vi "Configure Setpoint.vi"   [LabVIEW 2024, in "Bronkhorst FLOW-BUS.lvlib"]
doc: "Configures the setpoint value in the instrument. The setpoint is used to tell the PID controller in the instrument what the wanted amount of mass flow or pressure is."
uses:
  Bronkhorst FLOW-BUS.lvlib
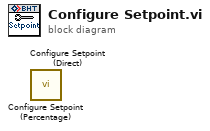
[diagram p0: block diagram]
diagram:
  n1 = call "Configure Setpoint (Percentage).vi"() -> ()  [unwired: 10 in, 2 out]
  n2 = call "Configure Setpoint (Direct).vi"() -> ()  [unwired: 10 in, 2 out]
